vi "Ocean Server OS4000 Series - Streaming.vi"(9 "Send Declination":bool, 10 "Declination Angle":i32, 11 "VISA resource name":refnum<visa-resource-name>) -> (1 "pitchAngle":dbl format="%#.3g", 2 "rollAngle":dbl format="%#.3g", 3 "compassHeading":dbl format="%#.3g")   [LabVIEW 2011]
doc: "Demonstrates how to stream messages from the instrument."
uses:
  Program Files (x86)/National Instruments/LabVIEW 2011/instr.lib/Ocean Server OS4000/Ocean Server OS4000.lvlib
panel:
  in  "Baud Rate":u32(ring)=19200 items=["4800"=4800, "9600"=9600, "14400"=14400, "19200"=19200, "38400"=38400, "57600"=57600, "115200"=115200]
  in  "Get only latest Data?":bool caption="Get Only Latest Data?"
  out "Error?":bool
  in  "Check Error":bool
  in  "Send Degauss":bool
  in  "Send Mount Orientation":bool
  in  "Send Filter Value":bool
  in  "Send Output Rate":bool
  in  "Degauss Every":i32
  in  "Mount Orientation (Default-Flat)":i32(ring)=1 items=["Standard-flat"=1, "Front"=2, "Port"=3, "Roof"=4, "Back"=5, "StarBoard"=6]
  in  "Analog to Digital Conversion":i32
  in  "Average Samples":i32
  in  "Output Rate":dbl
  in  "Stop":bool
  in  "Reset (True)":bool=TRUE
  in  "ID Query (False)":bool
  # "(c) 2009 National Instruments.  ALL RIGHTS RESERVED."
  # "Communication Configuration"
  # "Serial Configuration"
  # "Device Configuration"
  # "Filter Value"
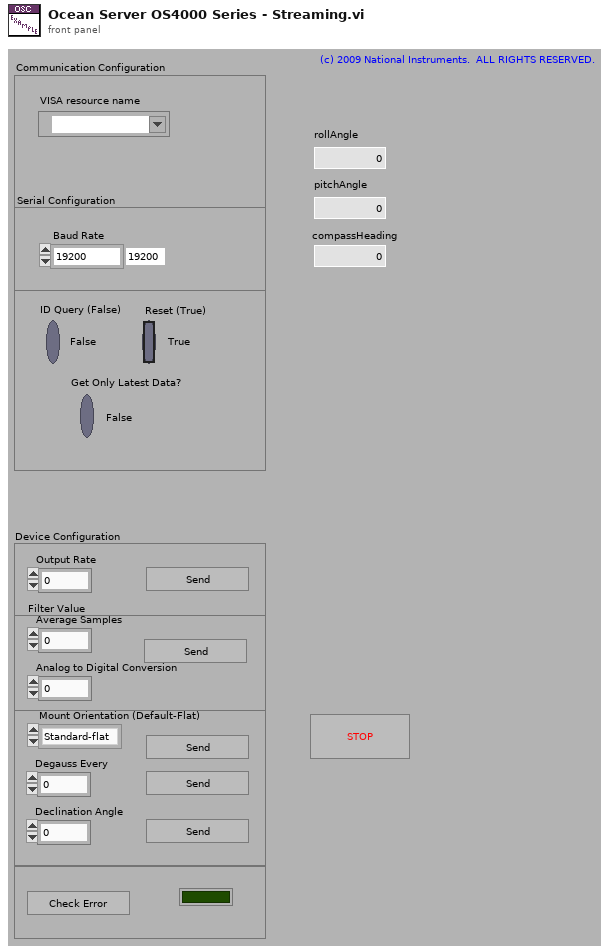
[diagram p1: front panel]
types:
  T1 = cluster{"Compass Heading":dbl, "pitch Angle":dbl, "roll Angle":dbl, "Temperature":dbl, "Depth":dbl, "Magnetic Field":dbl, "Magnetic Field X":dbl, "Magnetic Field Y":dbl, "Magnetic Field Z":dbl, "Acceleration":dbl, "Acceleration X":dbl, "Acceleration Y":dbl, "Gyro":dbl, "Gyro X":dbl, "Acceleration Z":dbl, "Gyro Y":dbl}
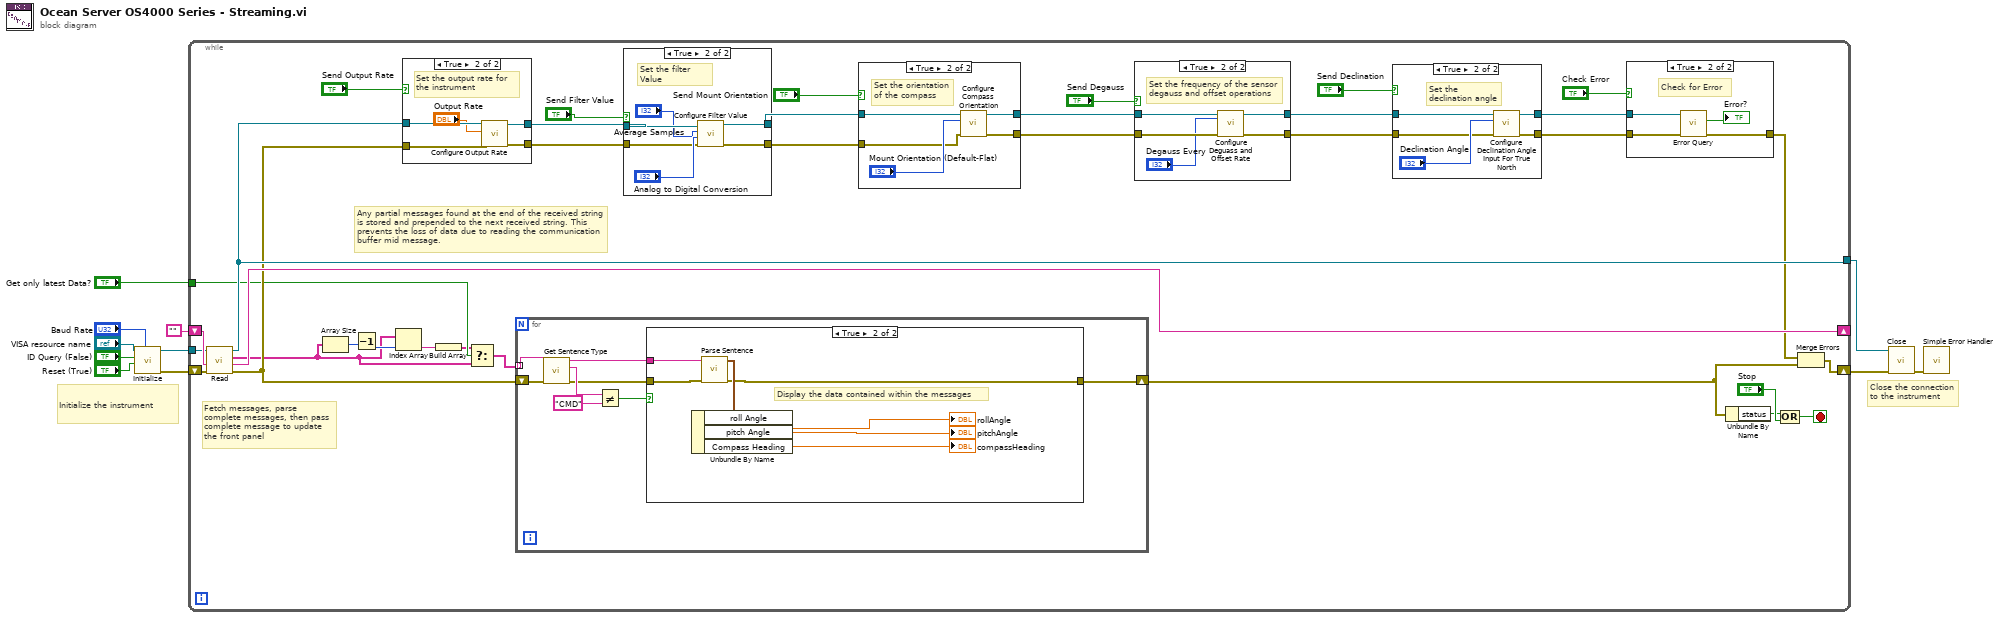
[diagram p0: block diagram]
diagram:
  # "Close the connection to the instrument"
  # "Initialize the instrument"
  n1 = call "Initialize.vi"("Baud Rate"="Baud Rate", "Reset (True)"="Reset (True)", "ID Query (False)"="ID Query (False)", "VISA resource name"="VISA resource name") -> ("error out"=w4:errorcluster, "VISA resource name out"=w3:refnum<visa-resource-name>)  [unwired: 6 in]
  n2 = while {
    shift-right: [w32] -> _
    shift-left: "" ("Remaining String") -> [w35]
    shift-right: [w21] -> w10
    shift-left: w4 -> [w33]
    tunnel: [w34] -> w11
    tunnel: w3 -> [w31]
    tunnel: "Get only latest Data?" -> [w18]
    stop <- w46 stop-if-true
    # "Any partial messages found at the end of the received string is stored and prepended to the next received string. This prevents the loss of data due to reading the communication buffer mid message."
    # "Fetch messages, parse complete messages, then pass  complete message to update the front panel"
    n3 = call "Read.vi"("error in (no error)"=w33, "Text to prepend to sentence"=w35, "VISA resource name"=w31) -> ("error out"=w27:errorcluster, "Remaining Sentence"=w32:string, "Ocean Server Sentences"=w13:string[], "VISA resource name out"=w34:refnum<visa-resource-name>)  [unwired: 5 in]
    n4 = Array Size(array=w13) -> (size(s)=w17:i32)
    n5 = Decrement(x=w17) -> (x-1=w16:i32)
    n6 = Index Array(array=w13, index=w16) -> (element=w15:string)
    n7 = case shown="True" "Send Output Rate" {
      tunnel: w34 -> [w98 w103]
      tunnel: [w98 w101] -> w43
      tunnel: [w97 w100] -> w30
      tunnel: w27 -> [w97 w99]
      frame False {
      }
      frame True {
        # "Set the output rate for the instrument"
        n8 = call "Configure Output Rate.vi"("Error in (no error)"=w99, "Output Rate ( 4 )"="Output Rate", "VISA resource name"=w103) -> ("Error out"=w100:errorcluster, "VISA resource out"=w101:refnum<visa-resource-name>)  [unwired: 7 in]
      }
    }
    n9 = Build Array(w15) -> (w14:string[])
    n10 = Select(t=w14, s=w18, f=w13) -> (s? t:f=w12:string[])
    n11 = for {
      tunnel: w12 -> [w54] mode=indexing
      shift-right: [w47] -> w19
      shift-left: w27 -> [w48]
      n12 = call "Get Sentence Type.vi"("error in (no error)"=w48, "Sentence In"=w54) -> ("error out"=w49:errorcluster, "Sentence Type"=w53:string, "Sentence Out"=w50:string)  [unwired: 7 in]
      n13 = Not Equal?(x=w53, y="CMD") -> (x != y?=w51:bool)
      n14 = case shown="True" w51 {
        tunnel: w50 -> [_ w59]
        tunnel: w49 -> [w55 w56]
        tunnel: [w55 w57] -> w47
        frame False {
          # "Front Panel isn't updated if the message received is not of the N1 type"
        }
        frame True {
          # "Display the data contained within the messages"
          n15 = call "Parse Sentence.vi"("error in (no error)"=w56, "Ocean Server Sentence"=w59) -> ("error out"=w57:errorcluster, "Values"=w58:T1)  [unwired: 8 in]
          n16 = Unbundle By Name(w58) -> ("roll Angle"=→"rollAngle":dbl, "pitch Angle"=→"pitchAngle":dbl, "Compass Heading"=→"compassHeading":dbl)
        }
      }
    }
    n17 = case shown="True" "Send Filter Value" {
      tunnel: w43 -> [w90 w96]
      tunnel: [w90 w93] -> w41
      tunnel: w30 -> [w89 w92]
      tunnel: [w89 w91] -> w29
      frame False {
      }
      frame True {
        # "Set the filter Value"
        n18 = call "Configure Filter Value.vi"("error in (no error)"=w92, "Filter Value for Analog to Digital Conversion ( 3 )"="Analog to Digital Conversion", "Averaging Value ( 4 )"="Average Samples", "VISA resource name"=w96) -> ("error out"=w91:errorcluster, "VISA resource out"=w93:refnum<visa-resource-name>)  [unwired: 6 in]
      }
    }
    n19 = case shown="True" "Send Mount Orientation" {
      tunnel: w41 -> [w83 w87]
      tunnel: [w83 w86] -> w39
      tunnel: w29 -> [w82 w85]
      tunnel: [w82 w84] -> w28
      frame False {
      }
      frame True {
        # "Set the orientation of the compass"
        n20 = call "Configure Compass Orientation.vi"("error in (no error)"=w85, "Mount Orientation ( Flat )"="Mount Orientation (Default-Flat)", "VISA resource name"=w87) -> ("error out"=w84:errorcluster, "VISA resource out"=w86:refnum<visa-resource-name>)  [unwired: 7 in]
      }
    }
    n21 = case shown="True" "Send Degauss" {
      tunnel: w39 -> [w76 w81]
      tunnel: [w76 w80] -> w38
      tunnel: [w75 w79] -> w37
      tunnel: w28 -> [w75 w78]
      frame False {
      }
      frame True {
        # "Set the frequency of the sensor degauss and offset operations"
        n22 = call "Configure Deguass and Offset Rate.vi"("error in (no error)"=w78, "Deguass and Offset Rate ( 1 )"="Degauss Every", "VISA resource name"=w81) -> ("error out"=w79:errorcluster, "VISA resource out"=w80:refnum<visa-resource-name>)  [unwired: 7 in]
      }
    }
    n23 = case shown="True" "Send Declination" {
      tunnel: w38 -> [w69 w73]
      tunnel: w37 -> [w68 w72]
      tunnel: [w69 w71] -> w24
      tunnel: [w68 w70] -> w23
      frame False {
      }
      frame True {
        # "Set the declination angle"
        n24 = call "Configure Declination Angle Input For True North.vi"("error in (no error)"=w72, "Declination Angle ( 0 degrees)"="Declination Angle", "VISA resource name"=w73) -> ("error out"=w70:errorcluster, "VISA resource out"=w71:refnum<visa-resource-name>)  [unwired: 7 in]
      }
    }
    n25 = case shown="True" "Check Error" {
      tunnel: w24 -> [_ w67]
      tunnel: w23 -> [w63 w66]
      tunnel: [w63 w64] -> w22
      frame False {
      }
      frame True {
        # "Check for Error"
        n26 = call "Error Query.vi"("error in (no error)"=w66, "VISA resource name"=w67) -> ("error out"=w64:errorcluster, "Error"=→"Error?":bool)  [unwired: 7 in, 1 out]
      }
    }
    n27 = Unbundle By Name(w19) -> ("status"=w26:bool)
    n28 = Compound Arithmetic op=OR(w26, "Stop") -> (w46:bool)
    n29 = Merge Errors(w22, w19) -> (w21:errorcluster)
  }
  n30 = call "Close.vi"("error in (no error)"=w10, "VISA resource name"=w11) -> ("error out"=w8:errorcluster)  [unwired: 9 in]
  n31 = call <vilib>:"Simple Error Handler.vi"("error in (no error)"=w8) -> ()  [unwired: 1 in, 8 out]
